vi "EventLog.Buffer.vi"(7 "action (get)":T6=enum."get", 8 "error in":errorcluster, 10 "Event in":T5={"ts"=0.0, "lev"=enum."Debug", "usr"=0, "src"=enum."All", "msg"=enum."Log out", "arg"=[]} {"ts" format="%<%X\n%x>T"}, 11 "Translations":string[](array[string])) -> (0 "error out":errorcluster, 1 "Translated Msg":string, 2 "data out":T1[](array[typedef]) {"ts" format="%<%X\n%x>T"}, 3 "Event out":T1={"ts"=0.0, "lev"=enum."Debug", "usr"=0, "src"=enum."All", "msg"=enum."Log out", "arg"=[], "msg_str"=""} {"ts" format="%<%X\n%x>T"})   [LabVIEW 2016]
uses:
  EventLog.Buffer.Action.ctl
  EventLog.Event.ctl
  EventLog.EventLevel.ctl
  EventLog.EventSource.ctl
  Translator/Translator.Message.ctl
  EventLog.EventGui.ctl
panel:
  out "Translations out":string[](array[string])
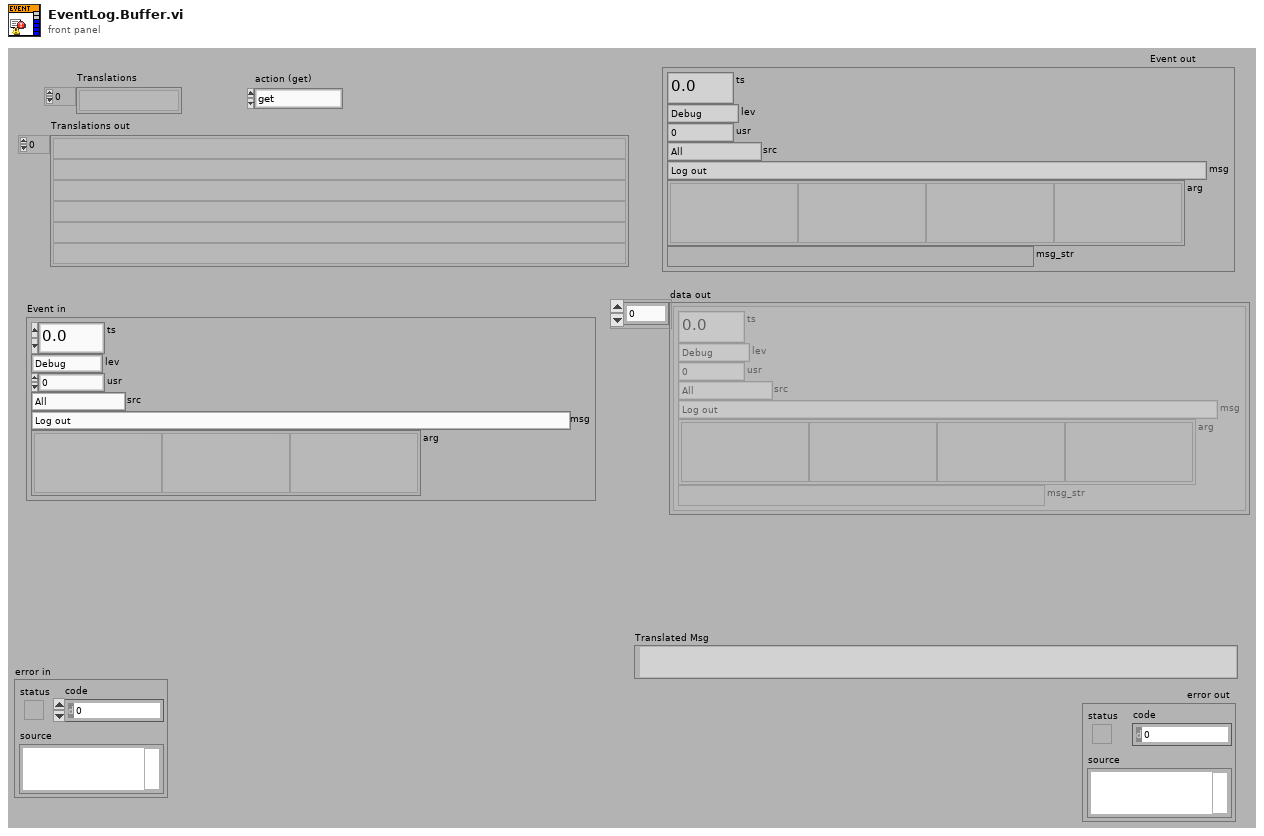
[diagram p1: front panel]
types:
  T1 = typedef "EventLog.EventGui.ctl" = cluster{"ts":dbl, "lev":T2, "usr":i32, "src":T3, "msg":T4, "arg":variant[], "msg_str":string}
  T2 = typedef "EventLog.EventLevel.ctl" = enum8{"Debug", "Info", "Warning", "Error"}
  T3 = typedef "EventLog.EventSource.ctl" = enum16{"All", "Gui", "Ref", "File", "Arch", "Seq", "CPX", "DB", "Laser", "Scan.P", "Scan.O"}
  T4 = typedef "Translator.Message.ctl" = enum16{"-", "Event confirmed", "Log out", "Log in", "Shutdown", "Cancel", "Start", "Begin time", "End time", "Duration", "Service Mode", "Ignore Results", "Serial Format", "On", "Off", "OK", "NOK", "NOK %s", "Home", "Work", "Close", "Open", "In progress...", "Missing", "Empty", "Hardware failure", "Initial", "Default", "Total", "Out of range", "Free disk space is below 1GB - contact technician", "Error %d >> %s", "Error %d >> %s >> %s", "Msg %d >> %s", "Laser msg %d %s", "Laser cmd error %s %d", "Laser cmd failed %s", "Laser cmd warning %s", "Laser disconnected", "Laser status %s", "Laser already started", "Laser job unkonwn %s", "Laser job missing %s", "Laser job select failure %s", "Unable to start laser printing (%s)", "Unable to stop laser printing (%s)", "Laser marking aborted", "Laser marking timeout", "Unable to reset Laser Interlock (%s)", "Unable to trigger Laser. Laser not ready (%s)", "Laser job '%s' coordinates not configured", "Starting %s", "Quitting %s", "Configured", "Initializing", "Quitting", "Loading", "Loaded %d results", "Loaded %d events", "Running", "Stopped", "Summary", "Laser", "Do you want to continue?", "Do you want to delete the configuration?", "The configuration is being used by an order. Unable to delete!", "Press confirm button", "Station is not based. Do you want to exit?", "Station requires changeover. Do you want to run the test?", "Test options are not set as default. Do you want to continue?", "Formatting of WabcoNo is disabled. Do you want to continue?", "Product not detected. Do you want to continue?", "Product scan failed. Do you want to continue?", "Calibration", "Log out?", "System", "All", "IDLE", "Translating...%s", "Not found", "Alarm %s", "Run", "Skip", "Abort", "Repeat", "Please wait...", "Database disconnected", "Database disconnected - changeover disabled!", "Login to database successful", "Login to database failed: %d; %s", "Unable to check the product status of reference %d - database disconnected", "Unable to set the product status of reference %d - database disconnected", "Variant file backup %s", "Read variant (%s)", "Result", "Station armed!", "Station requires changeover!", "Select reference number...", "EMERGENCY BUTTON - press Control button", "EMERGENCY DOOR - press Control button", "Resetting Emergency...", "Unable to reset safety circuit - Emergency Button pressed", "Unable to reset safety circuit - Emergency Side Door open", "Station not based", "Station based", "Station not empty", "Station basing...", "No order", "Press Start to begin new order", "Scanning new order", "Order NOK. Correct or scan again", "Order OK. Press Accept", "Order ready", "Revolver incorrect", "Fork incorrect", "Revolver missing", "Revolver empty", "Container missing", "Offline results", "Offline statistics", "Updating statistics %.1f %%", "DMC Configurator", "Door open", "Close the front door", "Press start button", "Done. Open the front door", "Running...", "Running...%.1f %%", "Pause %s", "Pause %s. NOK container missing", "Pause %s. OK container missing", "Pause %s. Revolver empty", "Pause %s. Revolver missing", "Pause %s. Revolver incorrect", "Pause %s. Fork missing", "Pause %s. Fork incorrect", "Pause %s. Too many failures", "Pause %s. Unloading failure", "Pause %s. One slot is not working", "Pause %s. Part order is done. Empty OK container", "Pause %s. Unable to move product to slot", "Pause %s. Unable to move back product pusher", "Pause %s. Unable to lift product", "Pause %s. Unable to move back product lifter", "Pause %s. Unable to move product arm to Work", "Pause %s. Unable to move product arm to NOK", "Pause %s. Unable to move product arm to OK", "Pause %s. Unable to unsuck the NOK product", "Pause %s. Unable to drop the NOK product", "Pause %s. Product OK missing", "Pause %s. Unable to unsuck the OK product", "Pause %s. Unable to drop the OK product", "Stopping...", "File '%s' is missing", "File '%s' is broken", "File '%s' is running", "Log file started (%s)", "Log file ended (%s)", "Log file stopped (%s)", "Log file ignored (%s)", "Log file exported (%s)", "Log file export failed (%s)", "Wrong serial number in log file", "Wrong reference number in log file", "Test steps are missing", "%s = %.3f", "Process param '%s' not found in DB", "Process param '%s' wrong order", "Process param '%s' value %.3f out of limits (%.3f; %.3f)", "Step%d param '%s' not found in DB", "Step%d param '%s' wrong order", "Step%d param '%s' value %.3f out of limits (%.3f; %.3f)", "Step%d EV '%s' not found in DB", "Step%d EV '%s' wrong order", "\"%s\" not found in DB", "\"%s\" wrong order", "\"%s\" value %.3f out of limits (%.3f; %.3f)", "\"%s\" not found in software", "Process init (%s)", "Process started", "Process restarted", "Process run", "Process done", "Process done - remove OK container", "Process aborted", "Process aborted at work", "Process aborted at home", "Process error", "Process error at home", "Process error at work", "Process close", "Process pause", "Process continue", "Process door open", "Process door close", "Process pause at slot %s due to %s", "Select plate from the order to process", "Do you want to start the process?", "Do you want to continue the process?", "There is unfinished order. Do you want to put the new order?", "Product %s %d OK", "Product %s %d NOK", "Unable to unload the slot %s. Product missing in the slot", "Unable to unload the slot %s. Product already in the arm", "Unable to accept the product as OK. Product missing in slot %s", "Unable to accept the product as OK. Product could not drop into the container at slot %s", "Unable to accept the product as NOK. Product could not drop into the container at slot %s", "Scan failed. Error %s", "Scan failed. Scanner disconnected", "Scan failed. Wrong Wabco number %d, limit (%d,%d)", "Scan failed. Wrong serial number %d, limit (%d,%d)", "Scan failed. Wrong date %d, limit (%d,%d)", "Scan failed. Wrong product wabco number %d (expected %d)", "Scan failed. Wrong product serial number %d (expected > 0)", "Scan OK %s", "Scan failed. Unable to determine table position (%s)", "Scan failed. Timeout", "Tune failed. Scanner disconnected", "Tune failed. Timeout", "%s = %d", "%s = %d->%d", "Unable to set %s = %.2f - Air Pressure Inside off", "Unable to set digital output '%s' = %d", "Unable to activate air pressure inside - timeout", "Unable to activate air pressure inside - aborted", "Unable to switch on Air Main Valve - Air Pressure Inlet off", "Unable to switch on Air Main Valve - Door open", "Unable to switch off Air Main Valve - timeout", "Unable to switch off Air Main Valve - aborted", "Unable to rotate Table - timeout", "Unable to rotate Table - aborted", "Unable to rotate Table - Product Move not in Home position", "Unable to rotate Table - Air Pressure Inside off", "Unable to rotate Table - Product Lift A not in Home position", "Unable to rotate Table - Product Lift B not in Home position", "Unable to rotate Table - unlock before movement timeout", "Unable to rotate Table - lock after movement timeout", "Unable to move Table Lock to %s position - timeout", "Unable to move Table Lock to %s position - aborted", "Unable to move Table Lock to %s position - Air Pressure Inside off", "Unable to move Table Lock to %s position - Table not in position", "Unable to move Product Lift A to %s position - timeout", "Unable to move Product Lift B to %s position - timeout", "Unable to move Product Lift A to %s position - aborted", "Unable to move Product Lift B to %s position - aborted", "Unable to move Product Lift A to %s position - Air Pressure Inside off", "Unable to move Product Lift B to %s position - Air Pressure Inside off", "Unable to move Product Lift A to %s position - Table not locked", "Unable to move Product Lift B to %s position - Table not locked", "Unable to move Product Lift A to %s position - Product Arm not in Work position", "Unable to move Product Lift B to %s position - Product Arm not in Work position", "Unable to set Product Suction Gripper %s to %s - timeout", "Unable to set Product Suction Gripper %s to %s - aborted", "Unable to set Product Suction Gripper %s to %s - Air Pressure Inside off", "Unable to set Product Suction Gripper %s to %s - Table slot unkown", "Unable to move Product Arm to %s position - timeout", "Unable to move Product Arm to %s position - aborted", "Unable to move Product Arm to %s position - Air Pressure Inside off", "Unable to move Product Arm to %s position - Product Lift A not in Home position", "Unable to move Product Arm to %s position - Product Lift B not in Home position", "Unable to move Product to %s position - timeout", "Unable to move Product to %s position - aborted", "Unable to move Product to %s position - Air Pressure Inside off", "Unable to move Product to %s position - Table not in position"}
  T5 = typedef "EventLog.Event.ctl" = cluster{"ts":dbl, "lev":T2, "usr":i32, "src":T3, "msg":T4, "arg":variant[]}
  T6 = typedef "EventLog.Buffer.Action.ctl" = enum16{"init", "re-init", "clear", "set translator", "add", "get", "get unsaved"}
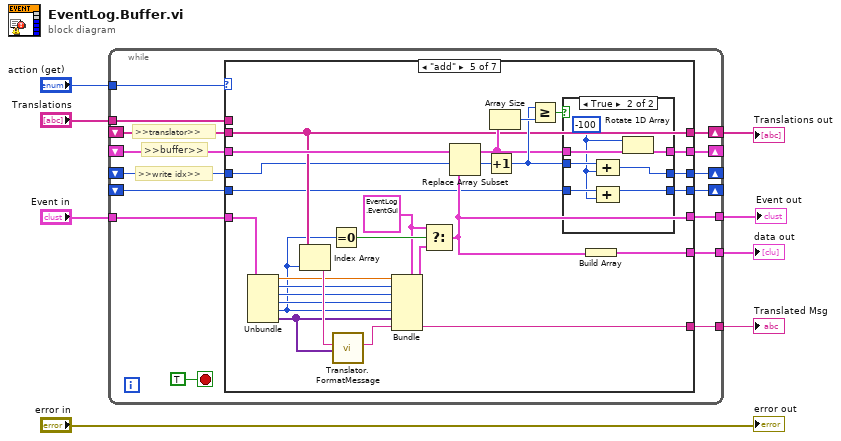
[diagram p0: block diagram]
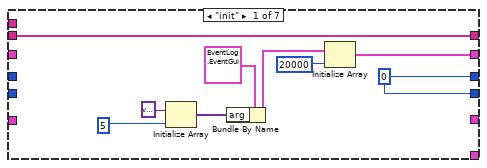
[diagram p2: hidden frame]
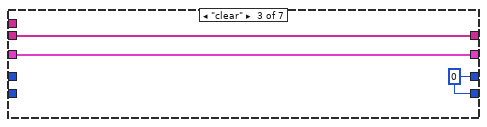
[diagram p4: hidden frame]
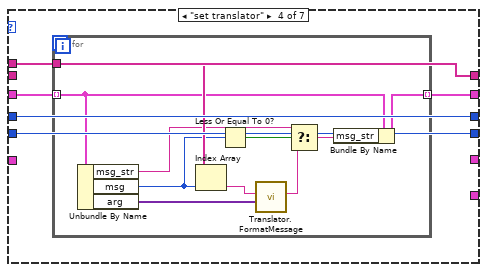
[diagram p5: hidden frame]
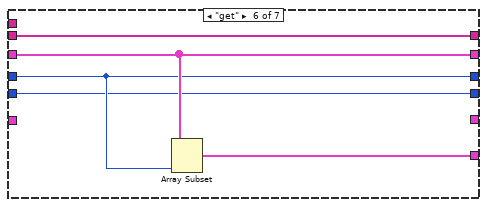
[diagram p7: hidden frame]
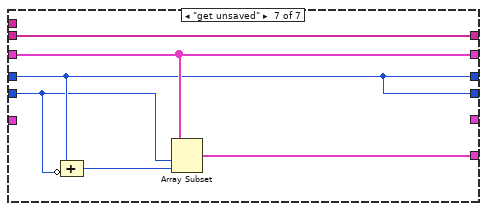
[diagram p8: hidden frame]
diagram:
  n1 = while {
    tunnel: "action (get)" -> [w22]
    tunnel: "Event in" -> [w21]
    shift-right: [w20] -> _
    shift-left: _ -> [w19]
    tunnel: [w18] -> w6
    shift-right: [w17] -> _
    shift-left: _ -> [w16]
    tunnel: "Translations" -> [w15]
    shift-right: [w14] -> w4
    shift-left: _ -> [w13]
    tunnel: [w12] -> w3
    tunnel: [w11] -> w2
    shift-right: [w10] -> _
    shift-left: _ -> [w9]
    stop <- TRUE stop-if-true
    # ">>write idx>>"
    # ">>translator>>"
    # ">>buffer>>"
    n2 = case shown="\"add\"" w22 {
      tunnel: w21 -> [_ _ _ _ w55 _ _]
      tunnel: [w31 w35 w38 w41 w73 w91 w97] -> w20
      tunnel: w19 -> [_ w35 w38 w42 w78 w91 w97]
      tunnel: [_ _ _ _ w68 w93 w99] -> w18
      tunnel: [w24 w33 w36 w43 w72 w90 w96] -> w17
      tunnel: w16 -> [_ w33 _ w43 w69 w90 w96]
      tunnel: w15 -> [_ _ _ w40 _ _ _]
      tunnel: [w26 w34 w37 w40 w71 w92 w98] -> w14
      tunnel: w13 -> [w26 w34 w37 _ w71 w92 w98]
      tunnel: [_ _ _ _ w60 _ _] -> w12
      tunnel: [_ _ _ _ w58 _ _] -> w11
      tunnel: [w24 w33 w36 w39 w56 w89 w96] -> w10
      tunnel: w9 -> [_ _ _ w39 w57 w89 w95]
      frame "init" {
        w24 = 0
        n3 = Initialize Array(variant ("Variant"), 5 ("dimension size")) -> (w27:variant[])
        n4 = Bundle By Name(cluster=T1 {"ts"=0.0, "lev"=enum."Debug", "usr"=0, "src"=enum."All", "msg"=enum."-", "arg"=[], "msg_str"=""} ("Event (GUI)"), "arg"=w27) -> (w30:T1)
        n5 = Initialize Array(w30, 20000 ("dimension size")) -> (w31:T1[])
      }
      frame "re-init" {
      }
      frame "clear" {
        w36 = 0
      }
      frame "set translator" {
        n6 = for {
          tunnel: w42 -> [w51] mode=indexing
          tunnel: w40 -> [w52]
          tunnel: [w50] -> w41 mode=indexing
          n7 = Unbundle By Name(w51) -> ("msg_str"=w44:string, "msg"=w48:T4, "arg"=w53:variant[])
          n8 = Index Array(array=w52, index=w48) -> (element=w49:string)
          n9 = Less Or Equal To 0?(x=w48) -> (x <= 0?=w47:bool)
          n10 = call "Translator.FormatMessage.vi"("Arguments"=w53, "Msg"=w49) -> ("Translated Msg"=w46:string)  [unwired: 9 in]
          n11 = Select(t=w44, s=w47, f=w46) -> (s? t:f=w45:string)
          n12 = Bundle By Name(cluster=w51, "msg_str"=w45) -> (w50:T1)
        }
      }
      frame "add" {
        w54 = T1 {"ts"=0.0, "lev"=enum."Debug", "usr"=0, "src"=enum."All", "msg"=enum."-", "arg"=[], "msg_str"=""} ("Event")
        n13 = Unbundle(w55) -> ("ts"=w65:dbl, "lev"=w64:T2, "usr"=w63:i32, "src"=w62:T3, "msg"=w61:T4, "arg"=w59:variant[])
        n14 = Index Array(array=w71, index=w61) -> (element=w70:string)
        n15 = Equal To 0?(x=w61) -> (x = 0?=w67:bool)
        n16 = call "Translator.FormatMessage.vi"("Arguments"=w59, "Msg"=w70) -> ("Translated Msg"=w60:string)  [unwired: 9 in]
        n17 = Bundle(cluster=w54, "ts"=w65, "lev"=w64, "usr"=w63, "src"=w62, "msg"=w61, "arg"=w59, "msg_str"=w60) -> (w66:T1)
        n18 = Select(t=w54, s=w67, f=w66) -> (s? t:f=w58:T1)
        n19 = Replace Array Subset(array=w78, new element=w58, index=w69) -> (w74:T1[])
        n20 = Increment(x=w69) -> (x+1=w75:i32)
        n21 = Array Size(array=w74) -> (size(s)=w77:i32)
        n22 = Greater Or Equal?(x=w75, y=w77) -> (x >= y?=w76:bool)
        n23 = case shown="True" w76 {
          tunnel: w75 -> [w79 w88]
          tunnel: w74 -> [w81 w87]
          tunnel: [w81 w86] -> w73
          tunnel: [w79 w85] -> w72
          tunnel: w57 -> [w80 w84]
          tunnel: [w80 w82] -> w56
          frame False {
          }
          frame True {
            w83 = -100 ("y")
            n24 = Compound Arithmetic op=ADD(w88, w83) -> (w85:i32)
            n25 = Compound Arithmetic op=ADD(w84, w83) -> (w82:i32)
            n26 = Rotate 1D Array(1:w87, 2:w83) -> (0:w86:T1[])
          }
        }
        n27 = Build Array(w58) -> (w68:T1[])
      }
      frame "get" {
        n28 = Array Subset(array=w91, length=w90) -> (w93:T1[])  [unwired: 1 in]
      }
      frame "get unsaved" {
        n29 = Compound Arithmetic op=ADD(w96, invert w95) -> (w94:i32)
        n30 = Array Subset(array=w97, index=w95, length=w94) -> (w99:T1[])
      }
    }
  }
  "data out" <- w6
  "Translations out" <- w4
  "Translated Msg" <- w3
  "Event out" <- w2
  "error out" <- "error in"
